vi "Array - Distinct.vi"() -> ()   [LabVIEW 2017, in "Transparent Assertions.Tests.lvlib" / "Assert Collection Distinct.lvlib"]
uses:
  Assert Collection Distinct.lvlib
  src/Transparent Assertions/Transparent Assertions.lvlib
panel:
  out "error out":errorcluster
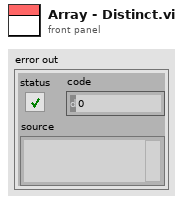
[diagram p1: front panel]
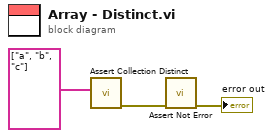
[diagram p0: block diagram]
diagram:
  n1 = call "Assert Collection Distinct.vi"("Collection"=string[] ["a", "b", "c"]) -> ("error out"=w3:errorcluster)  [unwired: 10 in]
  n2 = call "Assert Not Error.vi"("error in (no error)"=w3) -> ("error out"=→"error out":errorcluster)  [unwired: 10 in]
